vi "Localization.vi"(0 "OwningVIRefnum":refnum<vi>, 1 "ConfigFileRefnum":T1, 2 "Mode":enum16{"Read", "Write"}(ring), 3 "error in (no error)":errorcluster, 4 "DebugLOC":bool) -> (8 "error out":errorcluster)   [LabVIEW 2020, in "Localization_Tools.lvlib"]
uses:
  Localization_Tools.lvlib
  <vilib>/Utility/config.llb/Config Data RefNum.ctl
  <vilib>/Utility/config.llb/NI_LVConfig.lvlib
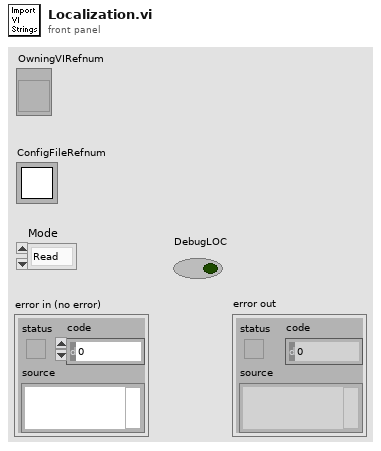
[diagram p1: front panel]
types:
  T1 = typedef "NI_LVConfig.lvlib/Config Data RefNum.ctl" = refnum<k1>
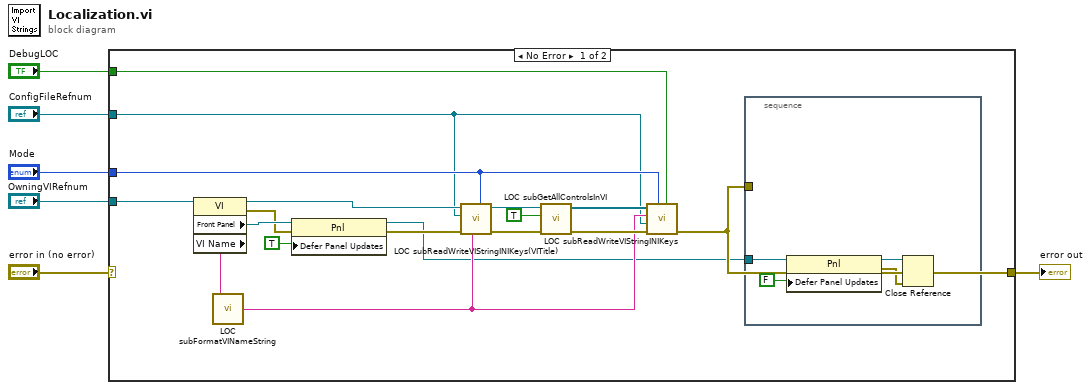
[diagram p0: block diagram]
diagram:
  n1 = case shown="No Error" "error in (no error)" {
    selector: "error in (no error)" -> [_ w29]
    tunnel: [w17 w29] -> w5
    tunnel: "Mode" -> [w11 _]
    tunnel: "ConfigFileRefnum" -> [w10 _]
    tunnel: "OwningVIRefnum" -> [w9 _]
    tunnel: "DebugLOC" -> [w8 _]
    frame No Error {
      n2 = property class="VI"(reference=w9) -> (reference out=w16:refnum<vi>, error out=w20:errorcluster, "Front Panel"=w22:refnum<vi>, "VI Name"=w23:string)  [unwired: 1 in]
      n3 = call "LOC subFormatVINameString.vi"("VIName"=w23) -> ("FormattedVIName"=w12:string)
      n4 = property class="Pnl"(reference=w22, error in=w20, "Defer Panel Updates"=TRUE) -> (reference out=w7:refnum<vi>, error out=w13:errorcluster)
      n5 = call "LOC subReadWriteVIStringINIKeys(VITitle).vi"("Mode"=w11, "VIName"=w12, "error in (no error)"=w13, "ConfigFileRefnum"=w10, "VIRefnum"=w16) -> ("error out"=w14:errorcluster, "dup VIRefnum"=w15:refnum<vi>)  [unwired: 3 in]
      n6 = call "LOC subGetAllControlsInVI.vi"("error in (no error)"=w14, "IgnoreCtrlsWithLeading \"_\""=TRUE ("IgnoreCtrlsWithLeading \"_\""), "VIRefnum"=w15) -> ("error out"=w19:errorcluster, "ControlRefnums"=w18:refnum<vi>[])  [unwired: 2 in, 1 out]
      n7 = call "LOC subReadWriteVIStringINIKeys.vi"("DebugLOC"=w8, "Mode"=w11, "error in (no error)"=w19, "ConfigFileRefnum"=w10, "VIName"=w12, "ControlRefnums"=w18) -> ("error out"=w17:errorcluster)  [unwired: 3 in]
      n8 = stacked-sequence {
        tunnel: w17 -> [_]
        tunnel: w7 -> [w25]
        frame #0 {
          n9 = property class="Pnl"(reference=w25, "Defer Panel Updates"=FALSE) -> (reference out=w27:refnum<vi>, error out=w26:errorcluster)  [unwired: 1 in]
          n10 = Close Reference(reference=w27, error in (no error)=w26) -> ()  [unwired: 1 out]
        }
      }
    }
    frame Error {
    }
  }
  "error out" <- w5
